vi "variable_son_globale.vi"() -> ()   [LabVIEW 2017]
panel:
  out "Son":waveform(dbl)[](graph)
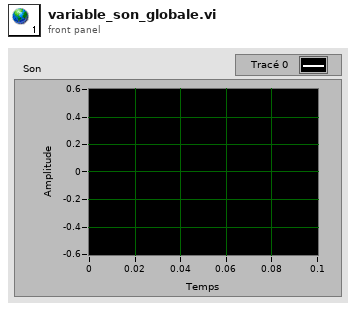
[diagram p1: front panel]
diagram:
